vi "niRFUtil RFHS Channelizer CreateNormalizeChannelsCfg CSG.vi"(0 "Channel Spec":T1={"freq in Hz"=TRUE, "Filter Type Hint"=enum."FFT (LTE)", "Hint Value"=0.5, "Channels"=[]} {"Channels"."Flags" items=["None"=0, "Force Fractional"=1, "Use Multistage"=2, "Use Pretrigger Data "=256, "Frequency Shift Only"=4]; "Channels"."fs" format="%#_8p"; "Channels"."fc" format="%#_6p"; "Channels"."stopBW" format="%#_6p"; "Channels"."passBW" format="%#_6p"; "Hint Value" format="%#_8p"}, 5 "fs [Hz]":dbl=1000000000.0 format="%#_6p", 11 "error in (no error)":errorcluster) -> (4 "Channel Spec (out)":T1={"freq in Hz"=TRUE, "Filter Type Hint"=enum."Auto", "Hint Value"=0.0, "Channels"=[]} {"Channels"."Flags" items=["None"=0, "Force Fractional"=1, "Use Multistage"=2, "Use Pretrigger Data "=256, "Frequency Shift Only"=4]; "Channels"."fs" format="%#_8p"; "Channels"."fc" format="%#_6p"; "Channels"."stopBW" format="%#_6p"; "Channels"."passBW" format="%#_6p"; "Hint Value" format="%#_8p"}, 15 "error out":errorcluster)   [LabVIEW 2015, in "niRFUtil.lvlib"]
uses:
  niRFUtil.lvlib
  Includes/niRFUtil RFHS Channelizer ChannelSpecification.ctl
  Includes/niRFUtil RFHS Channelizer FilterTypeHint.ctl
  Includes/niRFUtil RFHS Channelizer ChannelSpecificationBase.ctl
  Includes/niRFUtil RFHS Channelizer ChannelFlags.ctl
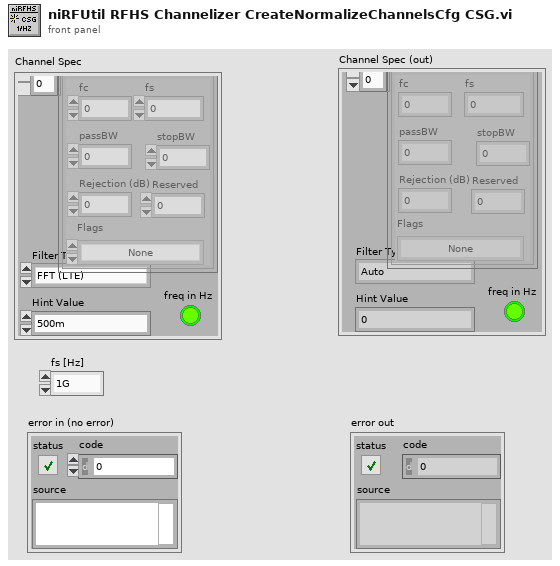
[diagram p1: front panel]
types:
  T1 = typedef "niRFUtil.lvlib/niRFUtil RFHS Channelizer ChannelSpecification.ctl" = cluster{"freq in Hz":bool, "Filter Type Hint":T2, "Hint Value":dbl, "Channels":T3[]}
  T2 = typedef "niRFUtil.lvlib/niRFUtil RFHS Channelizer FilterTypeHint.ctl" = enum16{"Auto", "FFT (LTE)", "FFT (WiFi)", "FFT (custom)"}
  T3 = typedef "niRFUtil.lvlib/niRFUtil RFHS Channelizer ChannelSpecificationBase.ctl" = cluster{"fc":dbl, "fs":dbl, "passBW":dbl, "stopBW":dbl, "Rejection (dB)":dbl, "Flags":T4, "Reserved":i32}
  T4 = typedef "niRFUtil.lvlib/niRFUtil RFHS Channelizer ChannelFlags.ctl" = u32
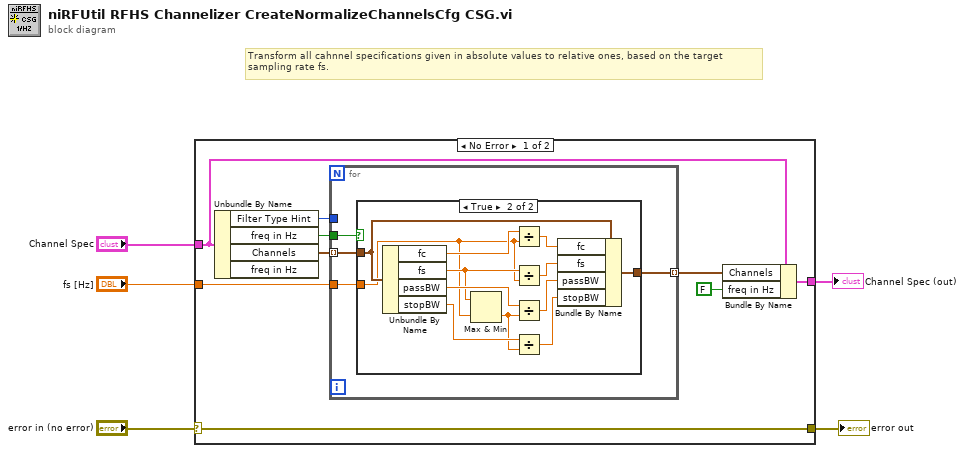
[diagram p0: block diagram]
diagram:
  # "Transform all cahnnel specifications given in absolute values to relative ones, based on the target \nsampling rate fs."
  n1 = case shown="No Error" "error in (no error)" {
    selector: "error in (no error)" -> [w6 w33]
    tunnel: "fs [Hz]" -> [w14 _]
    tunnel: "Channel Spec" -> [w13 w32]
    tunnel: [w12 w32] -> w3
    tunnel: [w6 w33] -> w1
    frame No Error {
      n2 = Unbundle By Name(w13) -> ("Filter Type Hint"=w10:T2, "freq in Hz"=w8:bool, "Channels"=w9:T3[])  [unwired: 1 out]
      n3 = for {
        tunnel: w14 -> [w16]
        tunnel: w9 -> [w17] mode=indexing
        tunnel: w8 -> [w18]
        tunnel: w10 -> [_]
        tunnel: [w15] -> w7 mode=indexing
        n4 = case shown="True" w18 {
          tunnel: w17 -> [w19 w28]
          tunnel: w16 -> [_ w21]
          tunnel: [w19 w24] -> w15
          frame False {
          }
          frame True {
            n5 = Unbundle By Name(w28) -> ("fc"=w31:dbl, "fs"=w22:dbl, "passBW"=w30:dbl, "stopBW"=w29:dbl)
            n6 = Max & Min(x=w22, y=w21) -> (min(x,y)=w20:dbl)  [unwired: 1 out]
            n7 = Divide(x=w31, y=w21) -> (x/y=w27:dbl)
            n8 = Divide(x=w22, y=w21) -> (x/y=w26:dbl)
            n9 = Divide(x=w30, y=w20) -> (x/y=w25:dbl)
            n10 = Divide(x=w29, y=w20) -> (x/y=w23:dbl)
            n11 = Bundle By Name(cluster=w28, "fc"=w27, "fs"=w26, "passBW"=w25, "stopBW"=w23) -> (w24:T3)
          }
        }
      }
      n12 = Bundle By Name(cluster=w13, "Channels"=w7, "freq in Hz"=FALSE) -> (w12:T1)
    }
    frame Error {
    }
  }
  "error out" <- w1
  "Channel Spec (out)" <- w3
